vi "Auto Select Model and Variant.vi"(8 "error in (no error)":errorcluster) -> (0 "error out":errorcluster, 1 "Ok":bool, 2 "Vaiant Selected":string, 3 "Model Selected":string)   [LabVIEW 2017]
uses:
  Database/Controls/DB Options.ctl
panel:
  in  "Cancel Button":bool
  in  "OK Button":bool
  in  "Variant":u16(ring)
  in  "Model":u16(ring)
  # "Select Model and Variant"
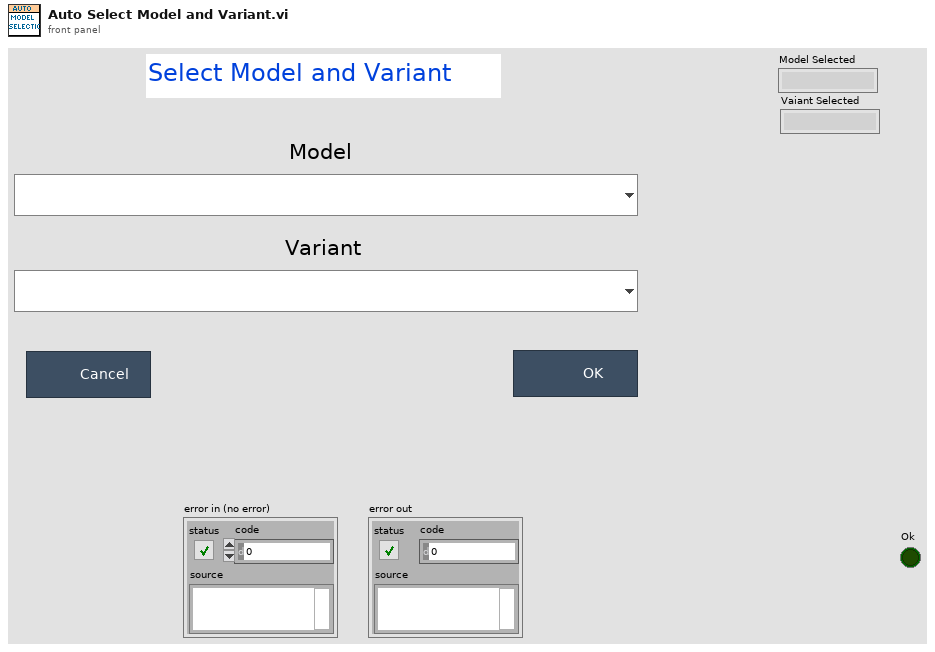
[diagram p1: front panel]
types:
  T1 = typedef "DB Options.ctl" = enum16{"Select", "Execute", "Special Q", "Insert", "Update", "Delete", "Open", "Close"}
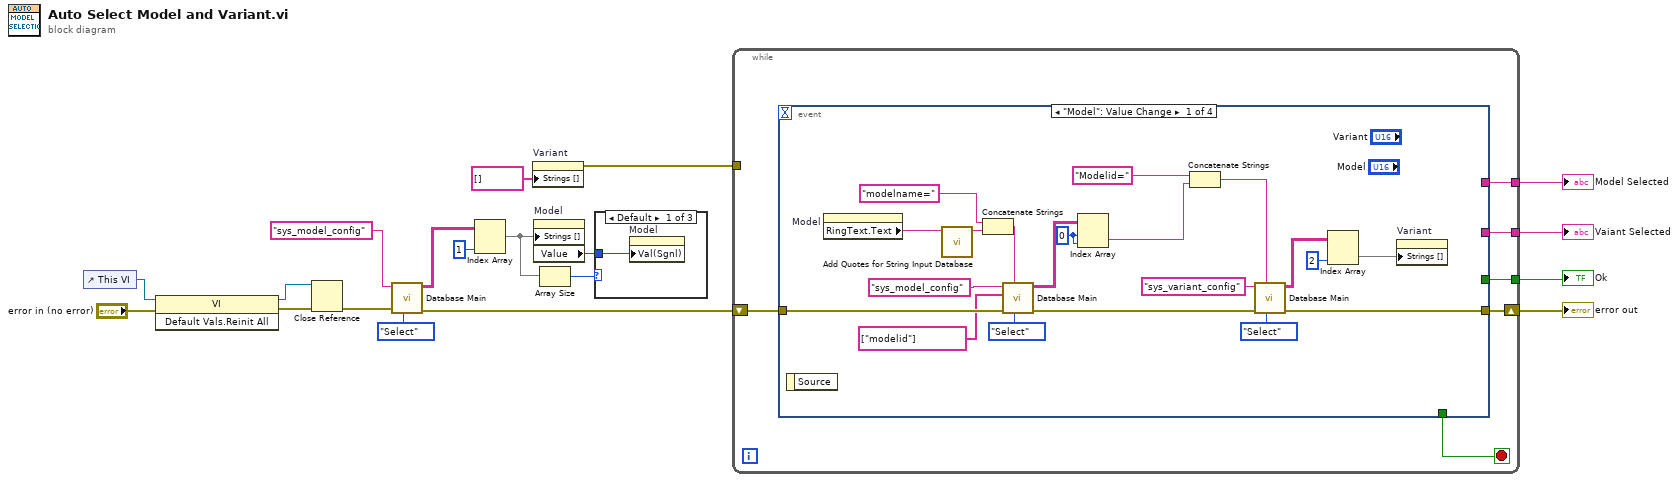
[diagram p0: block diagram]
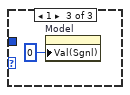
[diagram p3: hidden frame]
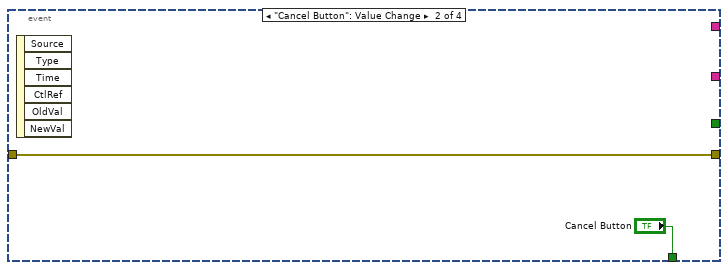
[diagram p4: hidden frame]
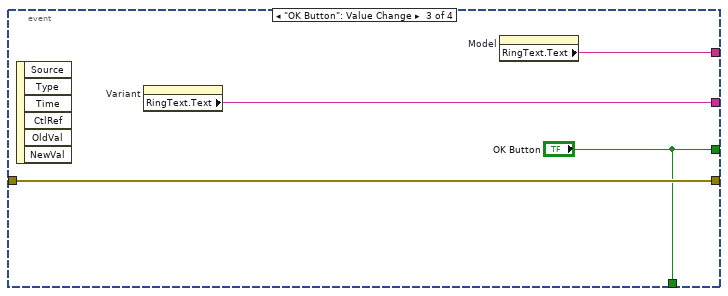
[diagram p5: hidden frame]
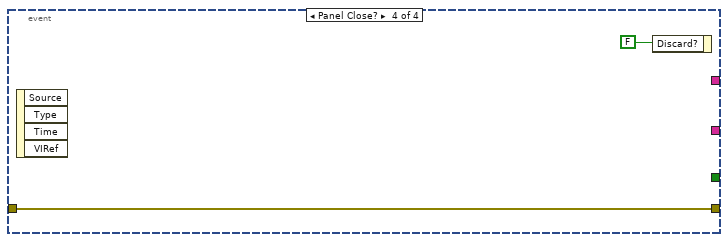
[diagram p6: hidden frame]
diagram:
  n1 = control-ref of="This VI"() -> (w8:refnum<vi>)
  n2 = invoke class="VI" method="Default Vals.Reinit All"(reference=w8, error in="error in (no error)") -> (reference out=w6:refnum<vi>, error out=w5:errorcluster)  [unwired: 1 in, 1 out]
  n3 = Close Reference(reference=w6, error in (no error)=w5) -> (error out=w4:errorcluster)
  n4 = call "Database Main.vi"("Option"=DB_Options."Select", "error in (no error)"=w4, "table Name/Query"="sys_model_config") -> ("error out"=w18:errorcluster, "Data"=w16:string[][])  [unwired: 6 in, 1 out]
  n5 = Index Array(array=w16, index (col)=1 ("disabled index (col)")) -> (element=w10:string[])  [unwired: 1 in]
  n6 = property on="Variant" class="Ring (strict)"("Strings []"=string[] []) -> (error out=w2:errorcluster)  [unwired: 2 in, 1 out]
  n7 = property on="Model" class="Ring (strict)"("Strings []"=w10) -> ("Value"=w1:u16)  [unwired: 2 in, 2 out]
  n8 = Array Size(array=w10) -> (size(s)=w9:i32)
  n9 = case shown="Default" w9 {
    tunnel: w1 -> [w20 _ _]
    frame Default {
      n10 = property on="Model" class="Ring (strict)"("Val(Sgnl)"=w20) -> ()  [unwired: 2 in, 2 out]
    }
    frame 0 {
    }
    frame 1 {
      n11 = property on="Model" class="Ring (strict)"("Val(Sgnl)"=u16 0 ("Value (Signaling)")) -> ()  [unwired: 2 in, 2 out]
    }
  }
  n12 = while {
    tunnel: [w25] -> w13
    tunnel: [w24] -> w12
    tunnel: [w23] -> w11
    shift-right: [w27] -> w19
    shift-left: w18 -> [w26]
    tunnel: w2 -> [_]
    stop <- w22 stop-if-true
    n13 = event shown="[0] \"Model\": Value Change" {
      selector: _ -> [_ _ _ _]
      dyn-events: _ -> [_ _ _ _]
      timeout: _ -> [_ _ _ _]
      tunnel: [w45 w49 w53 w54] -> w27
      tunnel: w26 -> [w39 w49 w53 w54]
      tunnel: [_ _ "OK Button" _] -> w25
      tunnel: [_ _ w52 _] -> w24
      tunnel: [_ _ w51 _] -> w23
      tunnel: [_ "Cancel Button" "OK Button" _] -> w22
      event "Model": Value Change {
        w32 = 0 ("index (row)")
        n14 = event-data() -> ()  [unwired: 1 in, 1 out]
        n15 = property on="Model" class="Ring (strict)"() -> ("RingText.Text"=w35:string)  [unwired: 2 in, 2 out]
        n16 = call "Add Quotes for String Input Database.vi"("String in"=w35) -> ("String Out"=w28:string)  [unwired: 10 in]
        n17 = Concatenate Strings("modelname=" ("Where"), w28) -> (w36:string)
        n18 = call "Database Main.vi"("Option"=DB_Options."Select", "Where"=w36, "error in (no error)"=w39, "Column Name"=string[] ["modelid"], "table Name/Query"="sys_model_config") -> ("error out"=w38:errorcluster, "Data"=w33:string[][])  [unwired: 4 in, 1 out]
        n19 = Index Array(array=w33, index (row)=w32, index (col)=w32) -> (element=w29:string)
        n20 = Concatenate Strings("Modelid=" ("Where"), w29) -> (w30:string)
        n21 = call "Database Main.vi"("Option"=DB_Options."Select", "Where"=w30, "error in (no error)"=w38, "table Name/Query"="sys_variant_config") -> ("error out"=w45:errorcluster, "Data"=w47:string[][])  [unwired: 5 in, 1 out]
        n22 = Index Array(array=w47, index (col)=2 ("disabled index (col)")) -> (element=w42:string[])  [unwired: 1 in]
        n23 = property on="Variant" class="Ring (strict)"("Strings []"=w42) -> ()  [unwired: 2 in, 2 out]
      }
      event "Cancel Button": Value Change {
        n24 = event-data() -> ()  [unwired: 1 in, 6 out]
      }
      event "OK Button": Value Change {
        n25 = event-data() -> ()  [unwired: 1 in, 6 out]
        n26 = property on="Variant" class="Ring (strict)"() -> ("RingText.Text"=w51:string)  [unwired: 2 in, 2 out]
        n27 = property on="Model" class="Ring (strict)"() -> ("RingText.Text"=w52:string)  [unwired: 2 in, 2 out]
      }
      event Panel Close? {
        n28 = event-data() -> ()  [unwired: 1 in, 4 out]
        n29 = event-data("Discard?"=FALSE) -> ()  [unwired: 1 in, 1 out]
      }
    }
  }
  "error out" <- w19
  "Ok" <- w13
  "Model Selected" <- w12
  "Vaiant Selected" <- w11
